vi "Read Response.vi"(8 "error in (no error)":errorcluster, 9 "Responses in":T1[](array[typedef]) {"Command" items=["Constant Speed Tracking"=8, "Echo"=55, "Error"=255, "Home"=1, "Limit Active"=9, "Manual Move Tracking"=10, "Move Absolute"=20, "Move at Constant Speed"=22, "Move Relative"=21, "Renumber"=2, "Restore Settings"=36, "Stop"=23]}, 10 "Partial Packet":string, 11 "VISA resource name":refnum<visa-resource-name>) -> (0 "error out":errorcluster, 1 "Responses out":T1[](array[typedef]) {"Command" items=["Constant Speed Tracking"=8, "Echo"=55, "Error"=255, "Home"=1, "Limit Active"=9, "Manual Move Tracking"=10, "Move Absolute"=20, "Move at Constant Speed"=22, "Move Relative"=21, "Renumber"=2, "Restore Settings"=36, "Stop"=23]}, 2 "Response":T1 {"Command" items=["Constant Speed Tracking"=8, "Echo"=55, "Error"=255, "Home"=1, "Limit Active"=9, "Manual Move Tracking"=10, "Move Absolute"=20, "Move at Constant Speed"=22, "Move Relative"=21, "Renumber"=2, "Restore Settings"=36, "Stop"=23]}, 3 "VISA resource name out":refnum<visa-resource-name>, 4 "Response Received?":bool)   [LabVIEW 2013, in "ZaberTSeries.lvlib"]
doc: "Reads a response packet from the serial port. If no response is waiting, Response just returns zeroes and Responses out equals Responses in. If Partial Packet is supplied, it is prepended to any input from the serial port."
uses:
  ZaberTSeries.lvlib
  Utility/Response.ctl
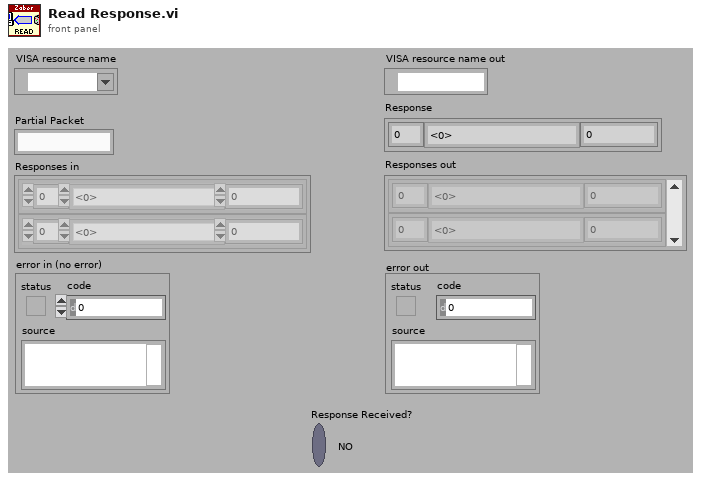
[diagram p1: front panel]
types:
  T1 = typedef "ZaberTSeries.lvlib/Response.ctl" = cluster{"Device Number":u8, "Command":u8, "Data":i32}
  T2 = cluster{"Device Number":u8, "Command":u8, "Data":u32}[]
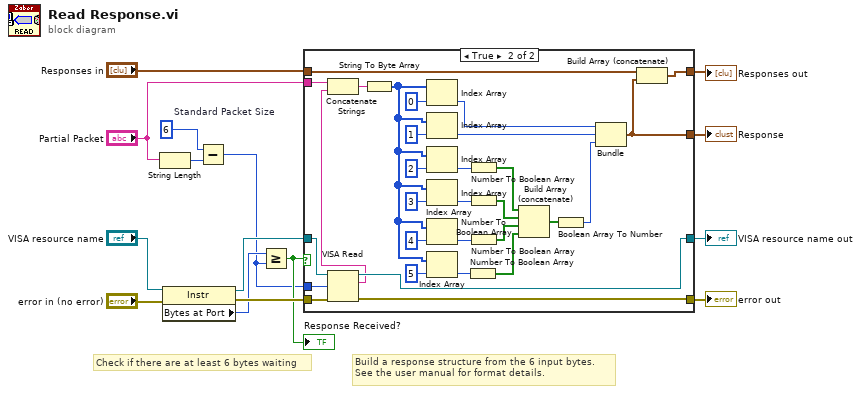
[diagram p0: block diagram]
diagram:
  w3 = 6  # Standard Packet Size
  # "Build a response structure from the 6 input bytes.\nSee the user manual for format details."
  # "Check if there are at least 6 bytes waiting"
  n1 = String Length(string="Partial Packet") -> (length=w2:i32)
  n2 = property class="Instr"(reference="VISA resource name", error in="error in (no error)") -> (reference out=w8:refnum<visa-resource-name>, error out=w9:errorcluster, "Bytes at Port"=w7:u32)
  n3 = Subtract(x=w3, y=w2) -> (x-y=w1:i32)
  n4 = Greater Or Equal?(x=w7, y=w1) -> (x >= y?=w6:bool)
  "Response Received?" <- w6
  n5 = case shown="True" w6 {
    tunnel: w8 -> [w16 w48]
    tunnel: [w18 w47] -> w13
    tunnel: w9 -> [w18 w46]
    tunnel: w1 -> [_ w26]
    tunnel: "Responses in" -> [w17 w24]
    tunnel: [w17 w25] -> w11
    tunnel: [w16 w23] -> w12
    tunnel: [_ w22] -> w5
    tunnel: "Partial Packet" -> [_ w19]
    frame False {
    }
    frame True {
      n6 = VISA Read(VISA resource name=w48, byte count=w26, error in (no error)=w46) -> (VISA resource name out=w23:refnum<visa-resource-name>, read buffer=w20:string, error out=w47:errorcluster)  [unwired: 1 out]
      n7 = Concatenate Strings(w19, w20) -> (w21:string)
      n8 = String To Byte Array(string=w21) -> (unsigned byte array=w39:u8[])
      n9 = Index Array(array=w39, index=0) -> (element=w29:u8)
      n10 = Index Array(array=w39, index=1) -> (element=w28:u8)
      n11 = Index Array(array=w39, index=2) -> (element=w38:u8)
      n12 = Index Array(array=w39, index=3) -> (element=w37:u8)
      n13 = Index Array(array=w39, index=4) -> (element=w36:u8)
      n14 = Index Array(array=w39, index=5) -> (element=w35:u8)
      n15 = Number To Boolean Array(number=w35) -> (Boolean array=w31:bool[])
      n16 = Number To Boolean Array(number=w38) -> (Boolean array=w34:bool[])
      n17 = Number To Boolean Array(number=w37) -> (Boolean array=w33:bool[])
      n18 = Number To Boolean Array(number=w36) -> (Boolean array=w32:bool[])
      n19 = Build Array (concatenate)(w34, w33, w32, w31) -> (w30:bool[])
      n20 = Boolean Array To Number(Boolean array=w30) -> (number=w27:u32)
      n21 = Bundle(w29, w28, w27) -> (w22:cluster{u8, u8, u32})  [unwired: 1 in]
      n22 = Build Array (concatenate)(w24, w22) -> (w25:T2)
    }
  }
  "error out" <- w13
  "Responses out" <- w11
  "VISA resource name out" <- w12
  "Response" <- w5
